vi "TRAFFIC LIGHT.vi"() -> ()   [LabVIEW 2020]
panel:
  in  "stop":bool
  in  "TIME YELLOW 2":dbl
  in  "TIME GREEN":dbl
  in  "TIME YELLOW":dbl
  out "SCREEN":dbl
  in  "TIME RED":dbl
  out "GREEN":bool
  out "YELLLOW":bool
  out "RED":bool
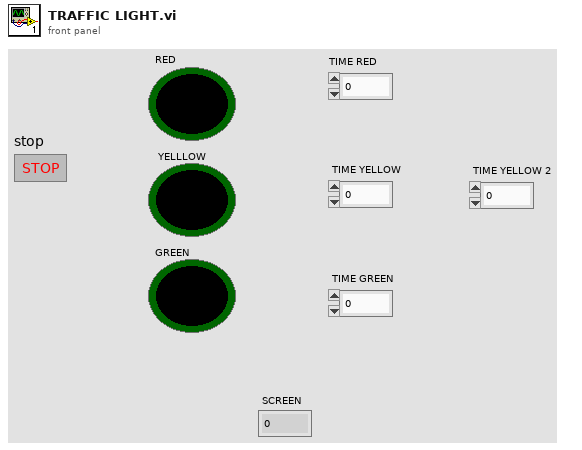
[diagram p1: front panel]
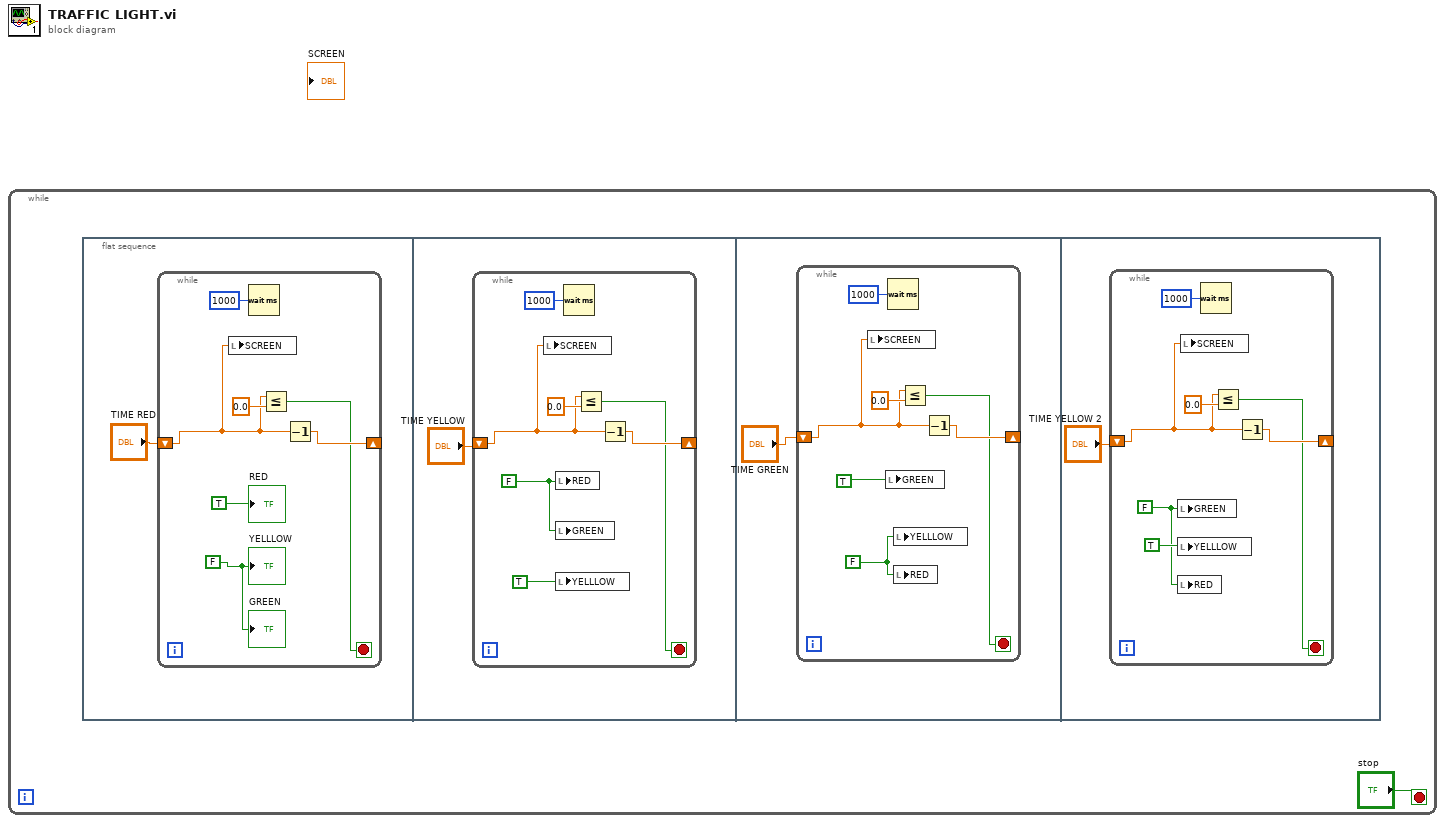
[diagram p0: block diagram]
diagram:
  n1 = while {
    stop <- "stop" stop-if-true
    n2 = flat-sequence {
      frame #0 {
        n3 = while {
          shift-right: [w9] -> _
          shift-left: "TIME RED" -> [w7]
          stop <- w6 stop-if-true
          w3 = FALSE
          n4 = local write "SCREEN"(w7) -> ()
          n5 = Wait (ms)(milliseconds to wait=u32 1000) -> ()  [unwired: 1 out]
          n6 = Less Or Equal?(x=w7, y=0.0) -> (x <= y?=w6:bool)
          n7 = Decrement(x=w7) -> (x-1=w9:dbl)
          "RED" <- TRUE
          "YELLLOW" <- w3
          "GREEN" <- w3
        }
      }
      frame #1 {
        n8 = while {
          shift-right: [w17] -> _
          shift-left: "TIME YELLOW" -> [w15]
          stop <- w14 stop-if-true
          w12 = FALSE
          n9 = local write "SCREEN"(w15) -> ()
          n10 = local write "RED"(w12) -> ()
          n11 = local write "GREEN"(w12) -> ()
          n12 = local write "YELLLOW"(TRUE) -> ()
          n13 = Wait (ms)(milliseconds to wait=u32 1000) -> ()  [unwired: 1 out]
          n14 = Less Or Equal?(x=w15, y=0.0) -> (x <= y?=w14:bool)
          n15 = Decrement(x=w15) -> (x-1=w17:dbl)
        }
      }
      frame #2 {
        n16 = while {
          shift-right: [w25] -> _
          shift-left: "TIME GREEN" -> [w23]
          stop <- w22 stop-if-true
          w19 = FALSE
          n17 = local write "SCREEN"(w23) -> ()
          n18 = local write "GREEN"(TRUE) -> ()
          n19 = Wait (ms)(milliseconds to wait=u32 1000) -> ()  [unwired: 1 out]
          n20 = local write "YELLLOW"(w19) -> ()
          n21 = local write "RED"(w19) -> ()
          n22 = Less Or Equal?(x=w23, y=0.0) -> (x <= y?=w22:bool)
          n23 = Decrement(x=w23) -> (x-1=w25:dbl)
        }
      }
      frame #3 {
        n24 = while {
          shift-right: [w33] -> _
          shift-left: "TIME YELLOW 2" -> [w31]
          stop <- w30 stop-if-true
          w27 = FALSE
          n25 = local write "GREEN"(w27) -> ()
          n26 = local write "YELLLOW"(TRUE) -> ()
          n27 = local write "RED"(w27) -> ()
          n28 = local write "SCREEN"(w31) -> ()
          n29 = Wait (ms)(milliseconds to wait=u32 1000) -> ()  [unwired: 1 out]
          n30 = Less Or Equal?(x=w31, y=0.0) -> (x <= y?=w30:bool)
          n31 = Decrement(x=w31) -> (x-1=w33:dbl)
        }
      }
    }
  }
